vi "KitBot-MOI-Frictionless.vi"() -> ()   [LabVIEW 2019]
uses:
  <vilib>/Rock Robotics/WPI/ThirdParty/JAS_Junk/TrajLib/Conv_Inches_Meters.vi
  <vilib>/Rock Robotics/WPI/ThirdParty/JAS_Junk/TrajLib/Trajectory_Library.lvlib
panel:
  out "KitBot MOI":dbl
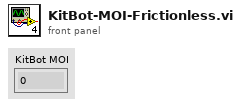
[diagram p1: front panel]
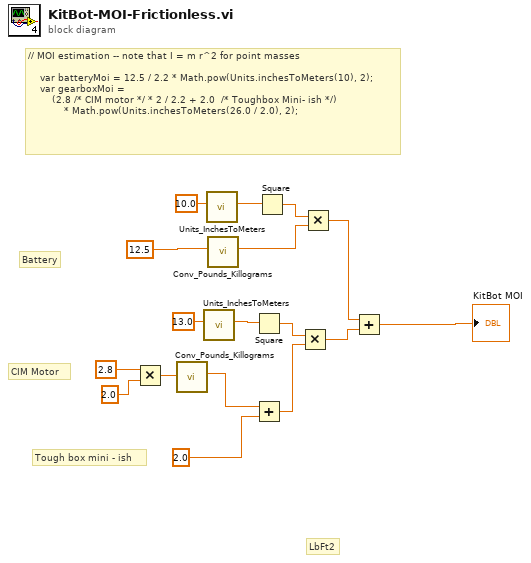
[diagram p0: block diagram]
diagram:
  # "LbFt2"
  # "Tough box mini - ish"
  # "Battery"
  # "CIM Motor"
  # "// MOI estimation -- note that I = m r^2 for point masses\n\n    var batteryMoi = 12.5 / 2.2 * Math.pow(Units.inchesToMeters(10), 2);\n    var gearboxMoi =\n        (2.8 /* CIM motor */ * 2 / 2.2 + 2.0 \t/* Toughbox Mini- ish */)\n            * Math.pow(Units.inchesToMeters(26.0 / 2.0), 2);"
  n1 = Multiply(x=2.8, y=2.0) -> (x*y=w2:dbl)
  n2 = call <vilib>:"Conv_Pounds_Killograms.vi"("Pounds"=w2) -> ("Killograms"=w1:dbl)  [unwired: 10 in]
  n3 = call <vilib>:"Units_InchesToMeters.vi"("Inches"=13.0) -> ("Meters"=w10:dbl)  [unwired: 10 in]
  n4 = call <vilib>:"Units_InchesToMeters.vi"("Inches"=10.0) -> ("Meters"=w14:dbl)  [unwired: 10 in]
  n5 = call <vilib>:"Conv_Pounds_Killograms.vi"("Pounds"=12.5 ("x")) -> ("Killograms"=w4:dbl)  [unwired: 10 in]
  n6 = Square(x=w10) -> (x^2=w9:dbl)
  n7 = Add(x=w1, y=2.0) -> (x+y=w8:dbl)
  n8 = Square(x=w14) -> (x^2=w13:dbl)
  n9 = Multiply(x=w9, y=w8) -> (x*y=w7:dbl)
  n10 = Multiply(x=w13, y=w4) -> (x*y=w6:dbl)
  n11 = Add(x=w6, y=w7) -> (x+y=→"KitBot MOI":dbl)
